vi "test-quintic-spline-00.vi"() -> ()   [LabVIEW 2019]
uses:
  <vilib>/Rock Robotics/WPI/ThirdParty/JAS_Junk/TrajLib/POSEwCURVATURE.ctl
  <vilib>/Rock Robotics/WPI/ThirdParty/JAS_Junk/TrajLib/POSE2D.ctl
  <vilib>/Rock Robotics/WPI/ThirdParty/JAS_Junk/TrajLib/TRANSLATION2D.ctl
  <vilib>/Rock Robotics/WPI/ThirdParty/JAS_Junk/TrajLib/ROTATION2D.ctl
  <vilib>/Rock Robotics/WPI/ThirdParty/JAS_Junk/TrajLib/Rotation_CreateAngle.vi
  <vilib>/Rock Robotics/WPI/ThirdParty/JAS_Junk/TrajLib/Translation_Create.vi
  <vilib>/Rock Robotics/WPI/ThirdParty/JAS_Junk/TrajLib/Util_CalcDist.vi
  <vilib>/Rock Robotics/WPI/ThirdParty/JAS_Junk/TrajLib/Trajectory_Library.lvlib
panel:
  out "XY Graph":cluster{dbl[], dbl[]}(graph)
  out "Numb\nWaypoints":i32
  out "All Interior \nwayPoints\nFound (True)":bool
  out "end rot = 0":dbl
  out "end y = 0":dbl
  out "end x = 0":dbl
  out "start rot = 0":dbl
  out "start y = 0":dbl
  out "start x = 0":dbl
  out "max dtheta < 0.0872":dbl
  out "max dy < 0.00127":dbl
  out "max dx  < 0.127":dbl
  out "Overall Error":errorcluster
  out "Elements":i32
  out "Create Spline Error":errorcluster
  out "SplinePoses\nWCurve":T1[](array[typedef]) {"POSE"."ROTATION"."SIN" format="%13.4f"; "POSE"."ROTATION"."COS" format="%13.4f"; "POSE"."ROTATION"."VALUE" format="%13.4f"; "POSE"."TRANSLATION"."Y" format="%14.3f"; "POSE"."TRANSLATION"."X" format="%14.3f"}
  out "Elapsed Time":dbl
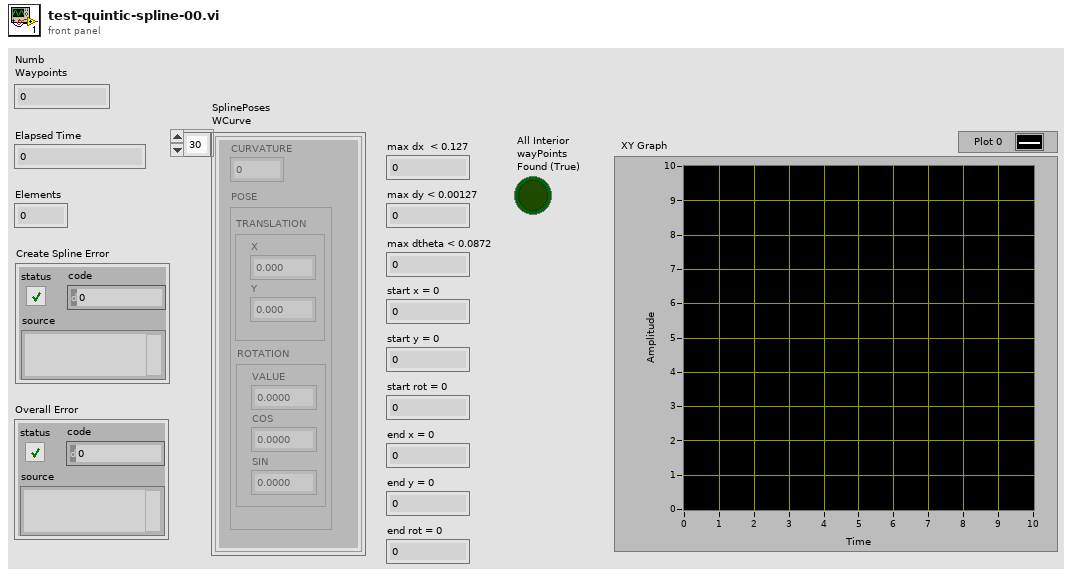
[diagram p1: front panel]
types:
  T1 = typedef "Trajectory_Library.lvlib/POSEwCURVATURE.ctl" = cluster{"CURVATURE":dbl, "POSE":T2}
  T2 = typedef "Trajectory_Library.lvlib/POSE2D.ctl" = cluster{"TRANSLATION":T3, "ROTATION":T4}
  T3 = typedef "Trajectory_Library.lvlib/TRANSLATION2D.ctl" = cluster{"X":dbl, "Y":dbl}
  T4 = typedef "Trajectory_Library.lvlib/ROTATION2D.ctl" = cluster{"VALUE":dbl, "COS":dbl, "SIN":dbl}
  T5 = typedef "Trajectory_Library.lvlib/SPLINE_CTRL_VECTOR.ctl" = cluster{"Xs":dbl[], "Ys":dbl[]}
  T6 = typedef "Trajectory_Library.lvlib/SPLINE.ctl" = cluster{"Degree":i32, "Coefficients":T7}
  T7 = typedef "NI_Matrix.lvlib/RealMatrix.ctl" = dbl[][]
  T8 = typedef "Trajectory_Library.lvlib/TWIST2D.ctl" = cluster{"dX":dbl, "dY":dbl, "dTHETA":dbl}
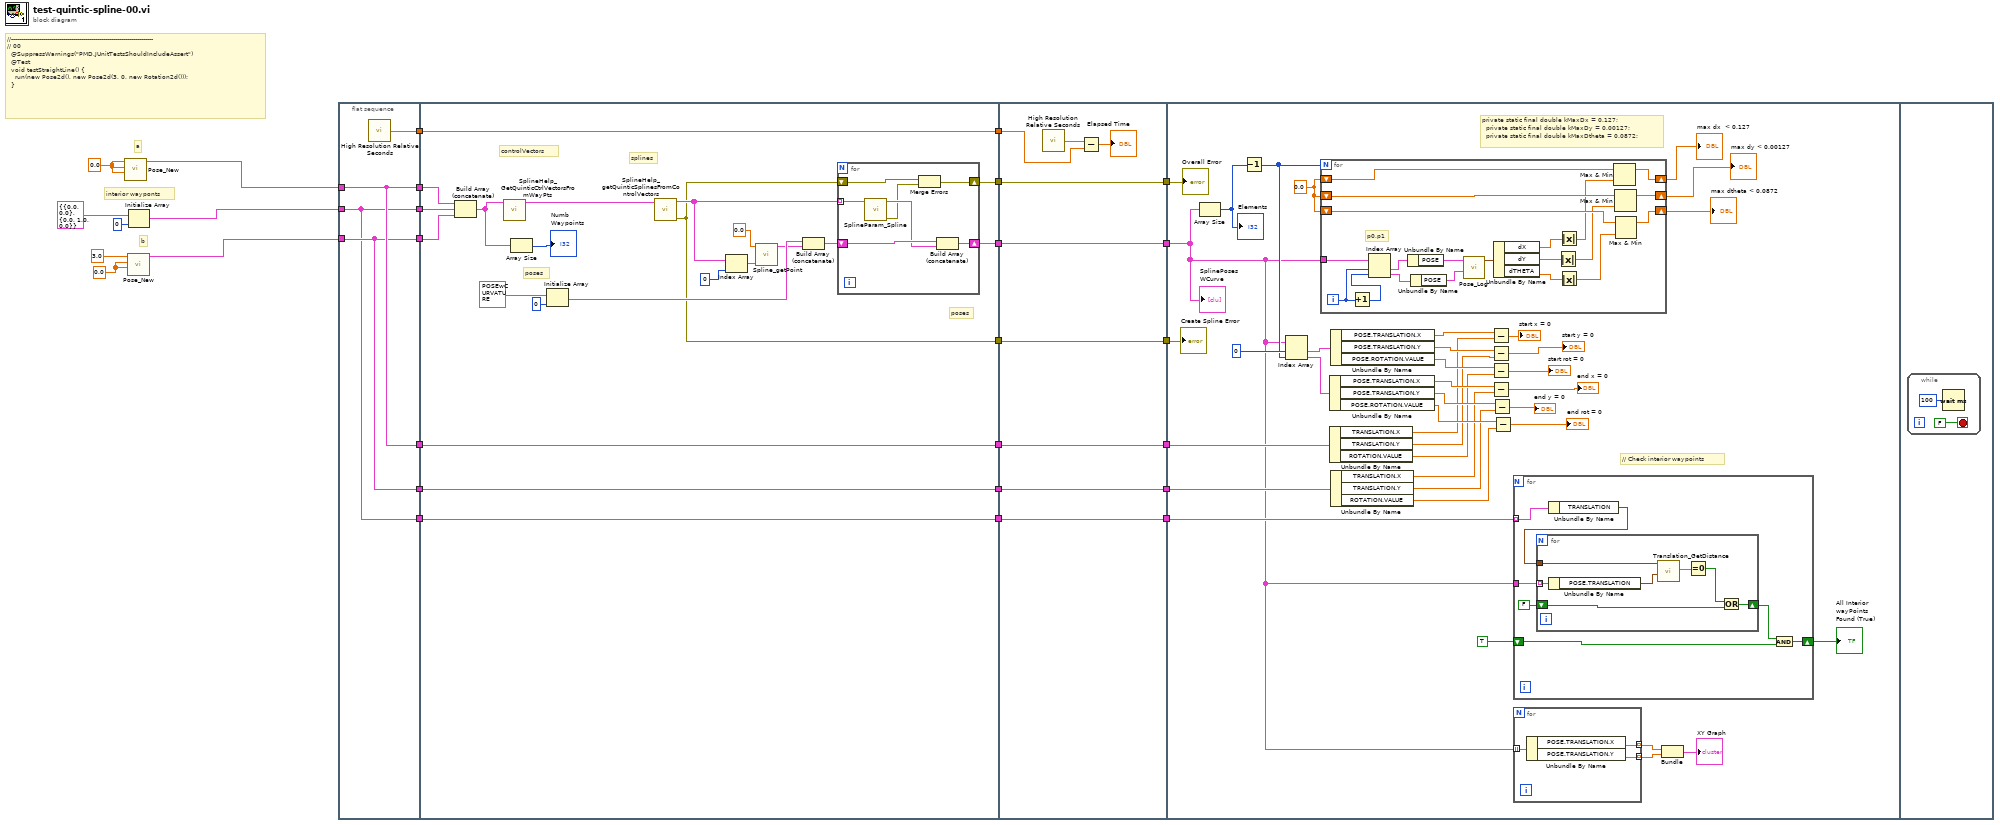
[diagram p0: block diagram]
diagram:
  w26 = 0.0 ("Y")
  w28 = 0.0 ("X")
  # "interior wayponts"
  # "b"
  # "a"
  # "//-----------------------------------------------------------------------\n// 00\n  @SuppressWarnings(\"PMD.JUnitTestsShouldIncludeAssert\")\n  @Test\n  void testStraightLine() {\n    run(new Pose2d(), new Pose2d(3, 0, new Rotation2d()));\n  }"
  n1 = call <vilib>:"Pose_New.vi"("Heading"=w28, "Y"=w28, "X"=w28) -> ("out POSe"=w25:T2)  [unwired: 8 in]
  n2 = call <vilib>:"Pose_New.vi"("Heading"=w26, "Y"=w26, "X"=3.0) -> ("out POSe"=w23:T2)  [unwired: 8 in]
  n3 = Initialize Array(T2 {"TRANSLATION"={"X"=0.0, "Y"=0.0}, "ROTATION"={"VALUE"=0.0, "COS"=1.0, "SIN"=0.0}} ("POSE"), 0 ("dimension size")) -> (w2:T2[])
  n4 = flat-sequence {
    tunnel: w25 -> [w31]
    tunnel: [w31] -> w24
    tunnel: w23 -> [w30]
    tunnel: [w30] -> w22
    tunnel: [w32] -> w21
    tunnel: [w31] -> w13
    tunnel: [w30] -> w10
    tunnel: [w29] -> w5
    tunnel: w2 -> [w29]
    tunnel: [w29] -> w1
    tunnel: w24 -> [w38]
    tunnel: w22 -> [w36]
    tunnel: [w54] -> w20
    tunnel: w21 -> [w54]
    tunnel: [w44] -> w19
    tunnel: [w43] -> w17
    tunnel: [w42] -> w15
    tunnel: w13 -> [w41]
    tunnel: [w41] -> w12
    tunnel: w10 -> [w40]
    tunnel: [w40] -> w9
    tunnel: [w39] -> w6
    tunnel: w5 -> [w39]
    tunnel: w1 -> [w35]
    tunnel: w20 -> [w70]
    tunnel: w19 -> [w69]
    tunnel: [w69] -> w18
    tunnel: w17 -> [w68]
    tunnel: [w68] -> w16
    tunnel: w15 -> [w67]
    tunnel: [w67] -> w14
    tunnel: w12 -> [w64]
    tunnel: [w64] -> w11
    tunnel: w9 -> [w63]
    tunnel: [w63] -> w8
    tunnel: [w62] -> w7
    tunnel: w6 -> [w62]
    tunnel: w18 -> [w72]
    tunnel: w16 -> [w108]
    tunnel: w14 -> [w107]
    tunnel: w11 -> [w101]
    tunnel: w8 -> [w100]
    tunnel: w7 -> [w77]
    frame #0 {
      n5 = call <vilib>:"High Resolution Relative Seconds.vi"() -> ("relative seconds"=w32:dbl)
    }
    frame #1 {
      # "poses"
      # "poses"
      # "splines"
      # "controlVectors"
      n6 = Build Array (concatenate)(w38, w35, w36) -> (w34:T2[])
      n7 = call <vilib>:"SplineHelp_GetQuinticCtrlVectorsFromWayPts.vi"("WayPoints"=w34) -> ("SplineControlVectors"=w37:T5[])  [unwired: 10 in]
      n8 = Array Size(array=w34) -> (size(s)=→"Numb\nWaypoints":i32)
      n9 = Initialize Array(T1 {"CURVATURE"=0.0, "POSE"={"TRANSLATION"={"X"=0.0, "Y"=0.0}, "ROTATION"={"VALUE"=0.0, "COS"=1.0, "SIN"=0.0}}} ("POSEwCURVATURE"), 0 ("dimension size")) -> (w48:T1[])
      n10 = call <vilib>:"SplineHelp_getQuinticSplinesFromControlVectors.vi"("ControlVectors"=w37) -> ("error out"=w43:errorcluster, "splines"=w45:T6[])  [unwired: 9 in]
      n11 = Index Array(array=w45, index=0) -> (element=w50:T6)
      n12 = call <vilib>:"Spline_getPoint.vi"("inputSPLINE"=w50, "Time"=0.0) -> ("POSEwCURVATURE"=w47:T1)  [unwired: 9 in]
      n13 = Build Array (concatenate)(w48, w47) -> (w46:T1[])
      n14 = for {
        shift-right: [w58] -> w44
        shift-left: w46 -> [w60]
        tunnel: w45 -> [w61] mode=indexing
        shift-right: [w56] -> w42
        shift-left: w43 -> [w57]
        n15 = call <vilib>:"SplineParam_Spline.vi"("inputSPLINE"=w61) -> ("error out"=w55:errorcluster, "outputPOSEwCURVATURE"=w59:T1[])  [unwired: 9 in]
        n16 = Merge Errors(w57, w55) -> (w56:errorcluster)
        n17 = Build Array (concatenate)(w60, w59) -> (w58:T1[])
      }
    }
    frame #2 {
      n18 = call <vilib>:"High Resolution Relative Seconds.vi"() -> ("relative seconds"=w65:dbl)
      n19 = Subtract(x=w65, y=w70) -> (x-y=→"Elapsed Time":dbl)
    }
    frame #3 {
      w105 = 0.0
      # "// Check interior waypoints"
      # "private static final double kMaxDx = 0.127;\n  private static final double kMaxDy = 0.00127;\n  private static final double kMaxDtheta = 0.0872;"
      n20 = Array Size(array=w72) -> (size(s)=w106:i32)
      "Elements" <- w106
      n21 = Decrement(x=w106) -> (x-1=w98:i32)
      n22 = Index Array(array=w72, index #1=0 ("index"), index #2=w98) -> (element #1=w97:T1, element #2=w96:T1)
      n23 = for {
        N: w98 -> [_]
        tunnel: w72 -> [w143]
        shift-right: [w134] -> w104
        shift-left: w105 -> [w131]
        shift-right: [w132] -> w102
        shift-left: w105 -> [w129]
        shift-right: [w133] -> w103
        shift-left: w105 -> [w130]
        i -> [w145]
        # "p0,p1"
        n24 = Increment(x=w145) -> (x+1=w144:i32)
        n25 = Index Array(array=w143, index #1=w145, index #2=w144) -> (element #1=w142:T1, element #2=w141:T1)
        n26 = Unbundle By Name(w142) -> ("POSE"=w140:T2)
        n27 = Unbundle By Name(w141) -> ("POSE"=w139:T2)
        n28 = call <vilib>:"Pose_Log.vi"("end POSE"=w139, "in POSE"=w140) -> ("out TWIST"=w138:T8)  [unwired: 9 in]
        n29 = Unbundle By Name(w138) -> ("dX"=w135:dbl, "dY"=w136:dbl, "dTHETA"=w137:dbl)
        n30 = Absolute Value(x=w136) -> (abs(x)=w127:dbl)
        n31 = Absolute Value(x=w135) -> (abs(x)=w128:dbl)
        n32 = Absolute Value(x=w137) -> (abs(x)=w126:dbl)
        n33 = Max & Min(x=w131, y=w128) -> (max(x,y)=w134:dbl)  [unwired: 1 out]
        n34 = Max & Min(x=w130, y=w127) -> (max(x,y)=w133:dbl)  [unwired: 1 out]
        n35 = Max & Min(x=w129, y=w126) -> (max(x,y)=w132:dbl)  [unwired: 1 out]
      }
      "max dx  < 0.127" <- w104
      "max dy < 0.00127" <- w103
      "max dtheta < 0.0872" <- w102
      n36 = Unbundle By Name(w96) -> ("POSE.TRANSLATION.X"=w92:dbl, "POSE.TRANSLATION.Y"=w91:dbl, "POSE.ROTATION.VALUE"=w90:dbl)
      n37 = Unbundle By Name(w101) -> ("TRANSLATION.X"=w89:dbl, "TRANSLATION.Y"=w88:dbl, "ROTATION.VALUE"=w87:dbl)
      n38 = Unbundle By Name(w97) -> ("POSE.TRANSLATION.X"=w95:dbl, "POSE.TRANSLATION.Y"=w94:dbl, "POSE.ROTATION.VALUE"=w93:dbl)
      n39 = Unbundle By Name(w100) -> ("TRANSLATION.X"=w86:dbl, "TRANSLATION.Y"=w85:dbl, "ROTATION.VALUE"=w84:dbl)
      n40 = Subtract(x=w95, y=w89) -> (x-y=→"start x = 0":dbl)
      n41 = Subtract(x=w94, y=w88) -> (x-y=→"start y = 0":dbl)
      n42 = Subtract(x=w93, y=w87) -> (x-y=→"start rot = 0":dbl)
      n43 = Subtract(x=w92, y=w86) -> (x-y=→"end x = 0":dbl)
      n44 = Subtract(x=w91, y=w85) -> (x-y=→"end y = 0":dbl)
      n45 = Subtract(x=w90, y=w84) -> (x-y=→"end rot = 0":dbl)
      n46 = for {
        tunnel: w77 -> [w113] mode=indexing
        tunnel: w72 -> [w118]
        shift-right: [w117] -> w75
        shift-left: TRUE -> [w116]
        n47 = Unbundle By Name(w113) -> ("TRANSLATION"=w112:T3)
        n48 = for {
          tunnel: w118 -> [w122] mode=indexing
          shift-right: [w125] -> w114
          shift-left: FALSE -> [w124]
          tunnel: w112 -> [w123]
          n49 = Unbundle By Name(w122) -> ("POSE.TRANSLATION"=w121:T3)
          n50 = call <vilib>:"Translation_GetDistance.vi"("other Translation"=w121, "In Translation"=w123) -> ("Distance"=w120:dbl)  [unwired: 9 in]
          n51 = Equal To 0?(x=w120) -> (x = 0?=w119:bool)
          n52 = Or(x=w119, y=w124) -> (x .or. y?=w125:bool)
        }
        n53 = And(x=w114, y=w116) -> (x .and. y?=w117:bool)
      }
      "All Interior \nwayPoints\nFound (True)" <- w75
      n54 = for {
        tunnel: [w111] -> w74 mode=indexing
        tunnel: [w110] -> w73 mode=indexing
        tunnel: w72 -> [w109] mode=indexing
        n55 = Unbundle By Name(w109) -> ("POSE.TRANSLATION.X"=w111:dbl, "POSE.TRANSLATION.Y"=w110:dbl)
      }
      n56 = Bundle(w74, w73) -> (→"XY Graph":cluster{dbl[], dbl[]})  [unwired: 1 in]
      "SplinePoses\nWCurve" <- w72
      "Create Spline Error" <- w108
      "Overall Error" <- w107
    }
    frame #4 {
      n57 = while {
        stop <- FALSE stop-if-true
        n58 = Wait (ms)(milliseconds to wait=u32 100) -> ()  [unwired: 1 out]
      }
    }
  }
